vi "histogram.vi"() -> ()   [LabVIEW 2025]
panel:
  in  "liczba cykli":i64
  in  "Sygnal":T1(ring)
  in  "phase":dbl
  in  "Amp":dbl
  in  "samples":i32=128
  in  "rozdzielczosc":dbl
  out "XY Graph":cluster{dbl[], i32[]}(graph)
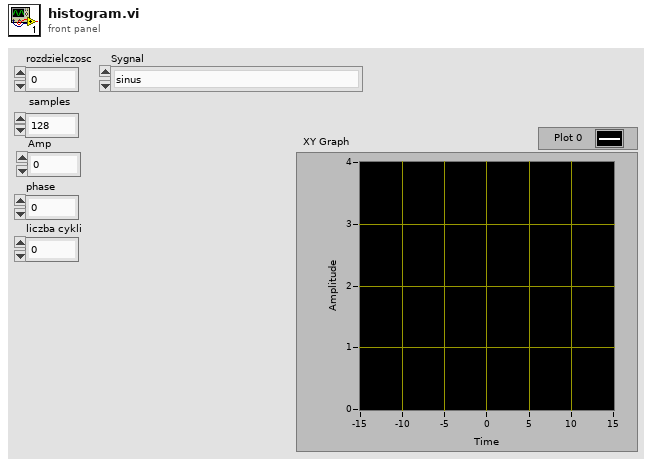
[diagram p1: front panel]
types:
  T1 = enum16{"sinus", "prostokat", "pila", "trojkat", "rozklad losowy", "rozklad normalny"}
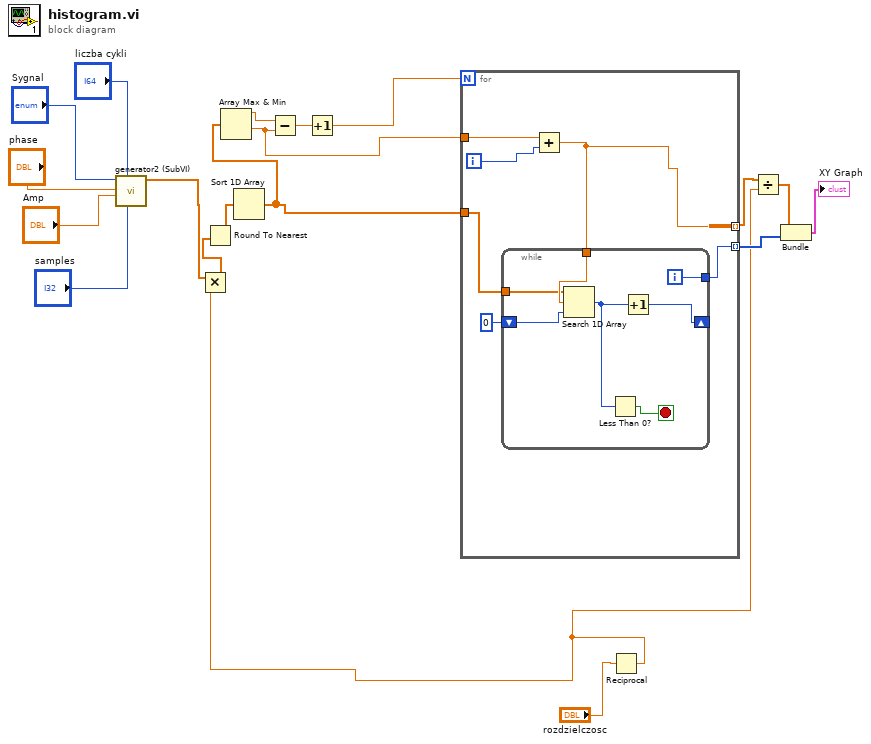
[diagram p0: block diagram]
diagram:
  n1 = call "generator2 (SubVI).vi"("samples"="samples", "liczba cykli"="liczba cykli", "Amp"="Amp", "phase"="phase", "Sygnal"="Sygnal") -> ("Gaussian noise pattern"=w6:dbl[])  [unwired: 6 in]
  n2 = Reciprocal(x="rozdzielczosc") -> (1/x=w7:dbl)
  n3 = Multiply(x=w6, y=w7) -> (x*y=w10:dbl[])
  n4 = Round To Nearest(number=w10) -> (nearest integer value=w9:dbl[])
  n5 = Sort 1D Array(array=w9) -> (sorted array=w15:dbl[])
  n6 = Array Max & Min(array=w15) -> (max value=w17:dbl, min value=w16:dbl)  [unwired: 2 out]
  n7 = Subtract(x=w17, y=w16) -> (x-y=w19:dbl)
  n8 = Increment(x=w19) -> (x+1=w18:dbl)
  n9 = for {
    N: w18 -> [_]
    tunnel: w16 -> [w25]
    tunnel: w15 -> [w24]
    tunnel: [w23] -> w14 mode=indexing
    tunnel: [w22] -> w12 mode=indexing
    i -> [w20]
    n10 = Add(x=w25, y=w20) -> (x+y=w22:dbl)
    n11 = while {
      tunnel: w22 -> [w31]
      tunnel: w24 -> [w30]
      shift-right: [w28] -> _
      shift-left: 0 -> [w29]
      tunnel: [w26] -> w23
      i -> [w26]
      stop <- w32 stop-if-true
      n12 = Search 1D Array(1D array=w30, element=w31, start index (0)=w29) -> (index of element=w27:i32)
      n13 = Less Than 0?(x=w27) -> (x < 0?=w32:bool)
      n14 = Increment(x=w27) -> (x+1=w28:i32)
    }
  }
  n15 = Divide(x=w12, y=w7) -> (x/y=w11:dbl[])
  n16 = Bundle(w11, w14) -> (→"XY Graph":cluster{dbl[], i32[]})  [unwired: 1 in]
